vi "checksum.vi"(9 "Ignore last term":bool, 11 "Array":u8[](array[numeric])) -> (3 "unsigned 8bit integer":u8)   [LabVIEW 2014]
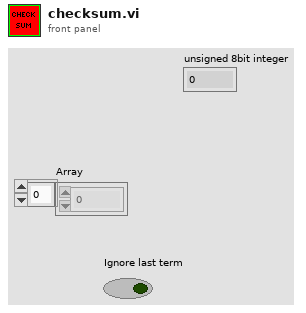
[diagram p1: front panel]
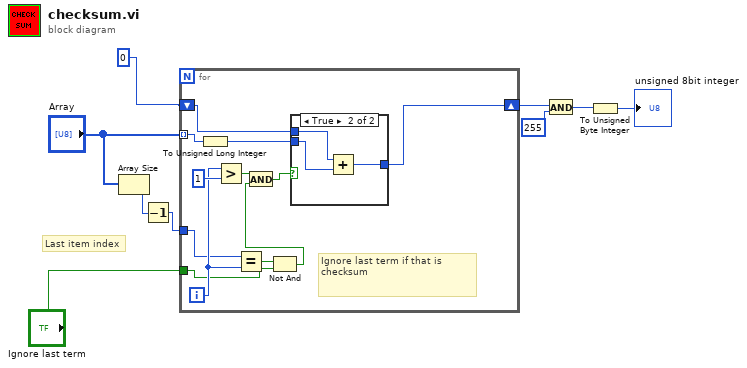
[diagram p0: block diagram]
diagram:
  # "Last item index"
  n1 = Array Size(array="Array") -> (size(s)=w2:i32)
  n2 = Decrement(x=w2) -> (x-1=w1:i32)
  n3 = for {
    tunnel: "Array" -> [w19] mode=indexing
    shift-right: [w17] -> w9
    shift-left: u32 0 -> [w20]
    tunnel: "Ignore last term" -> [w14]
    tunnel: w1 -> [w15]
    i -> [w16]
    # "Ignore last term if that is checksum"
    n4 = To Unsigned Long Integer(number=w19) -> (unsigned 32bit integer=w18:u32)
    n5 = Greater?(x=w16, y=1) -> (0:w12:bool)
    n6 = Equal?(x=w15, y=w16) -> (x = y?=w13:bool)
    n7 = Not And(1:w14, 2:w13) -> (0:w10:bool)
    n8 = And(x=w12, y=w10) -> (x .and. y?=w11:bool)
    n9 = case shown="True" w11 {
      tunnel: w20 -> [w22 w25]
      tunnel: w18 -> [_ w24]
      tunnel: [w22 w23] -> w17
      frame False {
      }
      frame True {
        n10 = Add(x=w25, y=w24) -> (x+y=w23:u32)
      }
    }
  }
  n11 = And(x=w9, y=u32 255) -> (x .and. y?=w7:u32)
  n12 = To Unsigned Byte Integer(number=w7) -> (unsigned 8bit integer=→"unsigned 8bit integer":u8)
